vi "RProp Update.vi"(10 "RProp Data":T1={"Empty Gradient"=[], "Gradient Register"=[], "Teach Coef Register"=[], "Current Gradient"=[], "# Vectors per Iteration"=2, "Teaching Set Ref"=refnum, "Validation Set Ref"=refnum, "Error Buffer"=[], "# Samples"=0, "Gradient Sign Running Value"=[]}, 11 "Neural Network In":refnum<class "Neural Network.lvclass">) -> (2 "RProp Data Out":T1={"Empty Gradient"=[], "Gradient Register"=[], "Teach Coef Register"=[], "Current Gradient"=[], "# Vectors per Iteration"=2, "Teaching Set Ref"=refnum, "Validation Set Ref"=refnum, "Error Buffer"=[], "# Samples"=0, "Gradient Sign Running Value"=[]}, 3 "Neural Network Out":refnum<class "Neural Network.lvclass">)   [LabVIEW 2015, in "Neural Network.lvclass"]
uses:
  Neural Network.lvclass
  Types/2D Array.ctl
  Types/RProp Algorithm.ctl
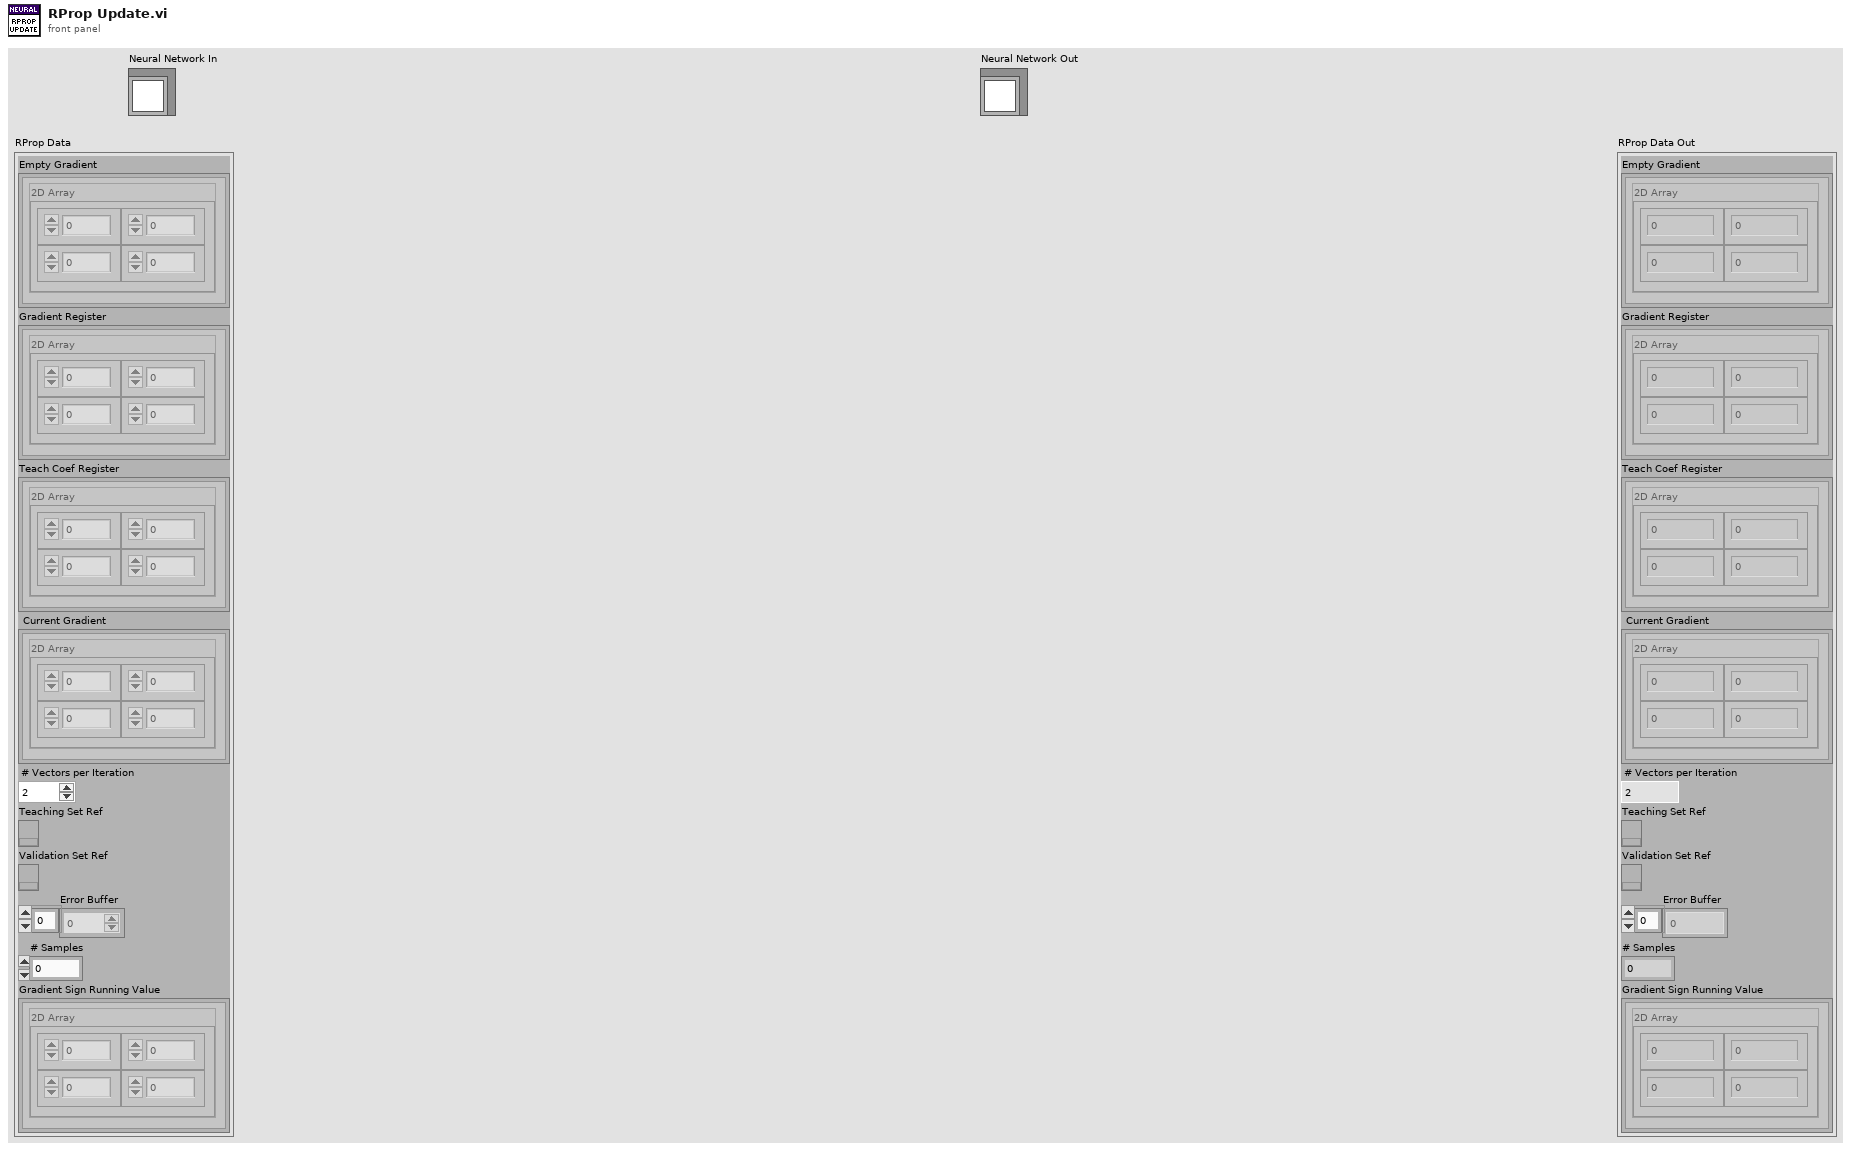
[diagram p1: front panel]
types:
  T1 = typedef "Neural Network.lvclass/RProp Algorithm.ctl" = cluster{"Empty Gradient":T2[], "Gradient Register":T2[], "Teach Coef Register":T2[], "Current Gradient":T2[], "# Vectors per Iteration":i64, "Teaching Set Ref":refnum<k34>, "Validation Set Ref":refnum<k34>, "Error Buffer":dbl[], "# Samples":i64, "Gradient Sign Running Value":T2[]}
  T2 = typedef "Neural Network.lvclass/2D Array.ctl" = cluster{"2D Array":sgl[][]}
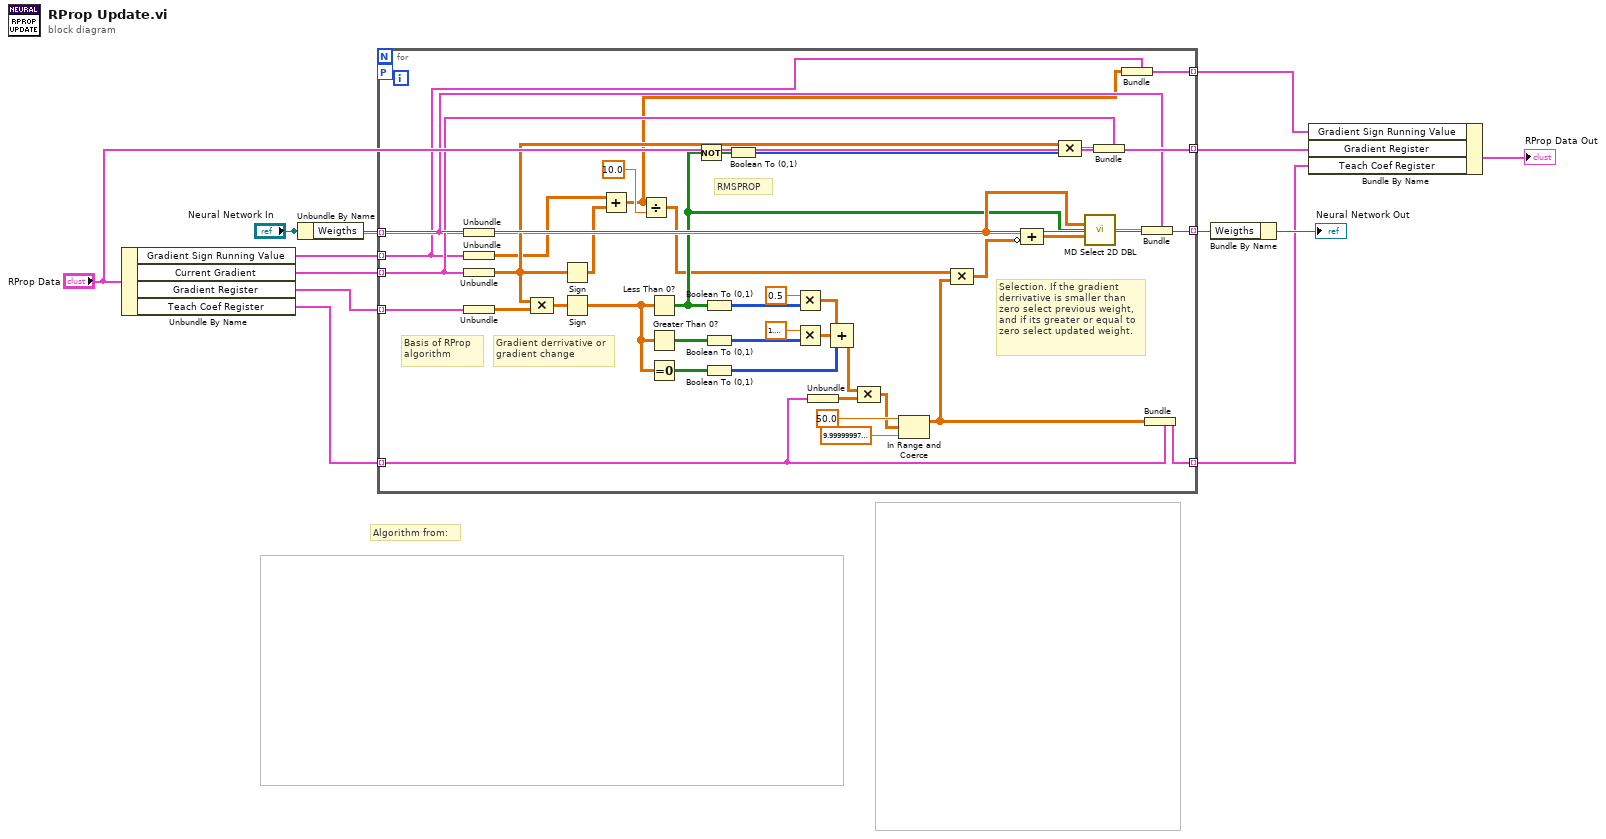
[diagram p0: block diagram]
diagram:
  # "Algorithm from:"
  n1 = Unbundle By Name("RProp Data") -> ("Gradient Sign Running Value"=w2:T2[], "Current Gradient"=w9:T2[], "Gradient Register"=w8:T2[], "Teach Coef Register"=w7:T2[])
  n2 = Unbundle By Name("Neural Network In") -> ("Weigths"=w10:T2[])
  n3 = for {
    tunnel: w10 -> [w27] mode=indexing
    tunnel: [w54] -> w11 mode=indexing
    tunnel: w9 -> [w28] mode=indexing
    tunnel: w8 -> [w53] mode=indexing
    tunnel: w7 -> [w25] mode=indexing
    tunnel: [w52] -> w4 mode=indexing
    tunnel: [w51] -> w5 mode=indexing
    workers-P: _ -> [_]
    tunnel: w2 -> [w16] mode=indexing
    tunnel: [w14] -> w1 mode=indexing
    # "RMSPROP"
    # "Selection. If the gradient\nderrivative is smaller than\nzero select previous weight,\nand if its greater or equal to\nzero select updated weight."
    # "Basis of RProp \nalgorithm"
    # "Gradient derrivative or\ngradient change"
    # "Iterate over the layers of the network and update the weigths"
    n4 = Unbundle(w27) -> ("2D Array"=w24:sgl[][])
    n5 = Unbundle(w16) -> ("2D Array"=w20:sgl[][])
    n6 = Unbundle(w28) -> ("2D Array"=w34:sgl[][])
    n7 = Unbundle(w53) -> ("2D Array"=w36:sgl[][])
    n8 = Compound Arithmetic op=MULTIPLY(w34, w36) -> (w43:sgl[][])
    n9 = Sign(1:w34) -> (0:w19:sgl[][])
    n10 = Sign(1:w43) -> (0:w45:sgl[][])
    n11 = Add(x=w20, y=w19) -> (x+y=w15:sgl[][])
    n12 = Divide(x=w15, y=sgl 10.0) -> (x/y=w17:sgl[][])
    n13 = Less Than 0?(x=w45) -> (x < 0?=w21:bool[][])
    n14 = Greater Than 0?(x=w45) -> (x > 0?=w50:bool[][])
    n15 = Equal To 0?(x=w45) -> (x = 0?=w39:bool[][])
    n16 = Not(x=w21) -> (.not. x?=w38:bool[][])
    n17 = Boolean To (0,1)(Boolean=w21) -> (0, 1=w26:i16[][])
    n18 = Boolean To (0,1)(Boolean=w50) -> (0, 1=w49:i16[][])
    n19 = Boolean To (0,1)(Boolean=w39) -> (0, 1=w40:i16[][])
    n20 = Boolean To (0,1)(Boolean=w38) -> (0, 1=w32:i16[][])
    n21 = Multiply(x=sgl 0.5, y=w26) -> (x*y=w30:sgl[][])
    n22 = Multiply(x=sgl 1.2, y=w49) -> (x*y=w29:sgl[][])
    n23 = Unbundle(w25) -> ("2D Array"=w48:sgl[][])
    n24 = Compound Arithmetic op=ADD(w30, w29, w40) -> (w44:sgl[][])
    n25 = Compound Arithmetic op=MULTIPLY(w44, w48) -> (w35:sgl[][])
    n26 = In Range and Coerce(upper limit=sgl 50.0, x=w35, lower limit=sgl 1e-06) -> (coerced(x)=w31:sgl[][])  [unwired: 1 out]
    n27 = Compound Arithmetic op=MULTIPLY(w17, w31) -> (w37:sgl[][])
    n28 = Compound Arithmetic op=ADD(w24, invert w37) -> (w23:sgl[][])
    n29 = Compound Arithmetic op=MULTIPLY(w34, w32) -> (w33:sgl[][])
    n30 = call "MD Select 2D DBL.vi"("First Array"=w24, "Condition"=w21, "Second Array"=w23) -> ("Resulting Array"=w22:sgl[][])  [unwired: 12 in]
    n31 = Bundle(cluster=w28, "2D Array"=w33) -> (w51:T2)
    n32 = Bundle(cluster=w16, "2D Array"=w15) -> (w14:T2)
    n33 = Bundle(cluster=w27, "2D Array"=w22) -> (w54:T2)
    n34 = Bundle(cluster=w25, "2D Array"=w31) -> (w52:T2)
  }
  n35 = Bundle By Name(cluster="Neural Network In", "Weigths"=w11) -> (→"Neural Network Out":refnum<class "Neural Network.lvclass">)
  n36 = Bundle By Name(cluster="RProp Data", "Gradient Sign Running Value"=w1, "Gradient Register"=w5, "Teach Coef Register"=w4) -> (→"RProp Data Out":T1)
